vi "Method.vi"(4 "Value":refnum<class "Abs_Complex Single Float.lvclass">) -> (1 "Result":refnum<class "Abs_Boolean.lvclass">)   [LabVIEW 2021, in "Not Equal 0_CPLX_SGL.lvclass"]
uses:
  Not Equal 0_CPLX_SGL.lvclass
  Abs_Types/Complex Single Float/Abs_Complex Single Float.lvclass
  Abs_Types/Boolean/Abs_Boolean.lvclass
  C:/TSA/LV_Abstract/Source/Functions/Support/Compare/One Term/CPLX_SGL/AbsComp_One Term_CPLX_SGL.lvclass
  C:/Program Files (x86)/National Instruments/LabVIEW 2021/vi.lib/TSA/Abstract Data Classes/Abs_Types/Boolean/Abs_Boolean.lvclass
  Support/Compare/One Term/CPLX_SGL/AbsComp_One Term_CPLX_SGL.lvclass/AbsComp_One Term_CPLX_SGL.ctl
  Support/Compare/One Term/CPLX_SGL/Properties/Write Numeric A.vi
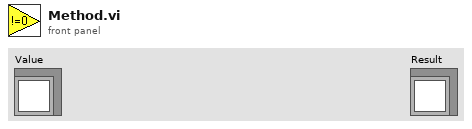
[diagram p1: front panel]
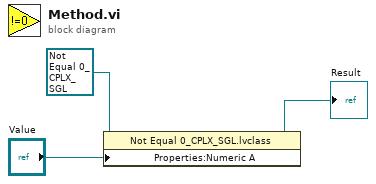
[diagram p0: block diagram]
diagram:
  n1 = property class="Not Equal 0_CPLX_SGL.lvclass"(reference=refnum<class "Not Equal 0_CPLX_SGL.lvclass"> refnum ("Greater 0_U64.lvclass"), "Properties:Numeric A"="Value") -> (reference out=→"Result":refnum<class "Not Equal 0_CPLX_SGL.lvclass">)  [unwired: 1 in, 1 out]
